vi "Simpletest.vi"() -> ()   [LabVIEW 2017]
panel:
  out "String":string
  in  "stop":bool
  out "Errors":string
  out "Version":string
  in  "VISA resource name":refnum<visa-resource-name>="ASRL30::INSTR"
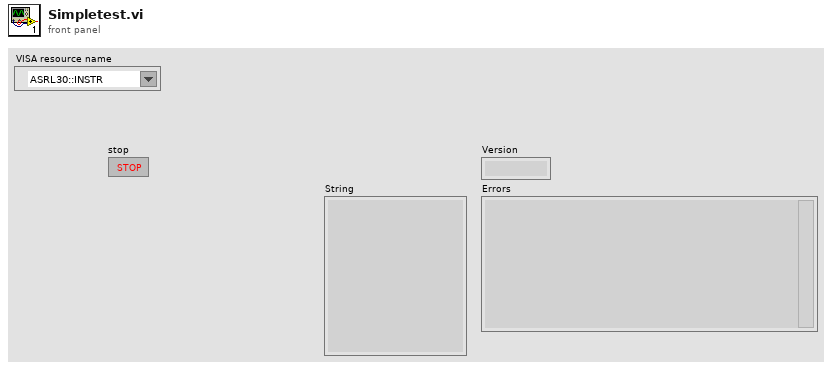
[diagram p1: front panel]
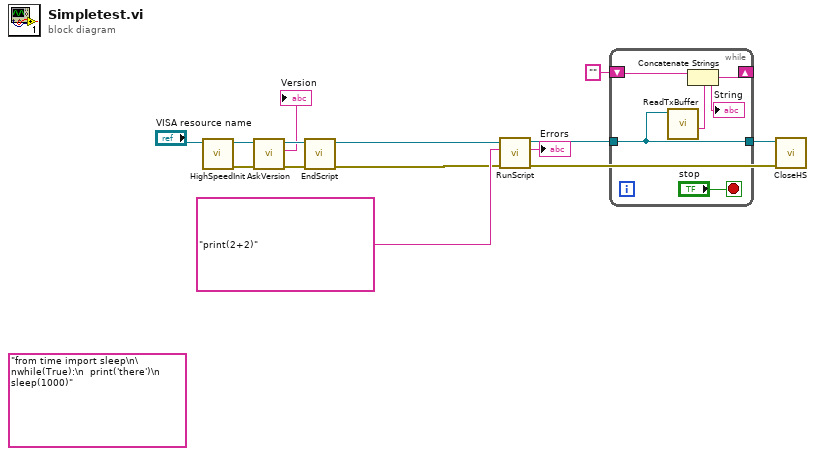
[diagram p0: block diagram]
diagram:
  (unwired) "from time import sleep\n\nwhile(True):\n  print('there')\n  sleep(1000)" ("header buffer")
  n1 = call "HighSpeedInit.vi"("VISA Refnum in"="VISA resource name") -> ("error out"=w13:errorcluster, "VISA Refnum out"=w12:refnum<visa-resource-name>)  [unwired: 9 in]
  n2 = call "AskVersion.vi"("error in"=w13, "VISA Refnum in"=w12) -> ("error out"=w11:errorcluster, "Version"=→"Version":string, "VISA Refnum out"=w10:refnum<visa-resource-name>)  [unwired: 7 in]
  n3 = call "EndScript.vi"("error in (no error)"=w11, "VISA Refnum in"=w10) -> ("error out"=w8:errorcluster, "VISA Refnum out"=w1:refnum<visa-resource-name>)  [unwired: 7 in, 1 out]
  n4 = call "RunScript.vi"("error in"=w8, "script"="print(2+2)" ("header buffer"), "VISA Refnum in"=w1) -> ("error out"=w6:errorcluster, "Tx"=→"Errors":string, "VISA Refnum out"=w3:refnum<visa-resource-name>)  [unwired: 6 in]
  n5 = while {
    tunnel: [w18] -> w4
    tunnel: w3 -> [w18]
    shift-right: [w15] -> _
    shift-left: "" -> [w17]
    stop <- "stop" stop-if-true
    n6 = call "ReadTxBuffer.vi"("VISA Refnum in"=w18) -> ("Tx Buffer"=w16:string)  [unwired: 7 in, 3 out]
    n7 = Concatenate Strings(w17, w16) -> (w15:string)
    "String" <- w15
  }
  n8 = call "CloseHS.vi"("error in (no error)"=w6, "VISA Refnum in"=w4) -> ()  [unwired: 10 in]
